vi "Point Shoot Example - MultipleSpectro.vi"(8 "Error in (no error)":errorcluster, 9 "Y":dbl, 10 "X":dbl, 11 "Method":enum16{"init", "run", "end"}(ring)) -> (0 "Error out":errorcluster)   [LabVIEW 2016]
doc: "Example of a measurement VI to be used in the \"Point & Shoot\" tool in Follow Me mode as external VI.\n\nThis example performs multiple bias spectroscopy measurements after each movement.\n\n- Nanonis Programming Interface -"
uses:
  Nanonis Prog Interface.lvlib
panel:
  in  "# Spectro. per point":i32=4
  # "Example of a measurement VI to be used in the \"Point & Shoot\" section of Follow Me mode as external VI.\n\nThis example performs multiple spectroscopy measurement after the movement in the Follow Me mode when Point & Shoot is enabled.\n\nTo use it, set up the bias spectroscopy module to record the desired channels and set all other spectroscopy parameters. Then, set up the experiments on Point & Shoot section to use this VI as \"external VI\".\n \n\"Point & Shoot\" will first (before starting the measurements) call the external VI with the \"init\" method, passing X and Y coordinates of the point.\nThen, for the measurements, the external VI will be called with the \"run\" method.\nAfter the last measurement, the external VI will be called with the \"end\" method."
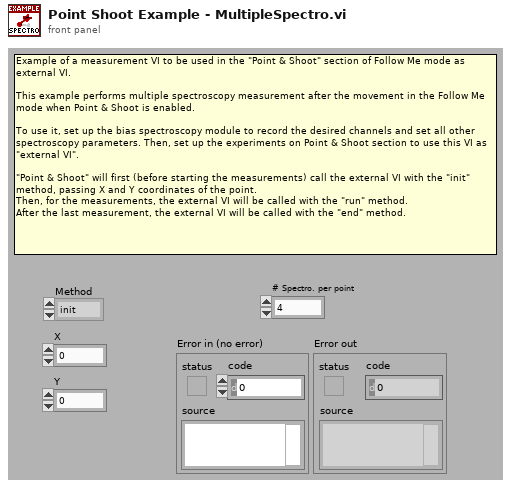
[diagram p1: front panel]
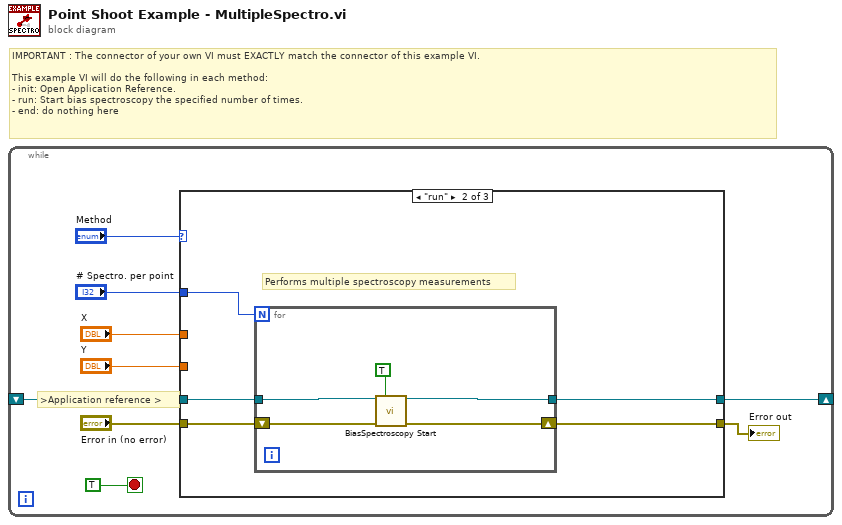
[diagram p0: block diagram]
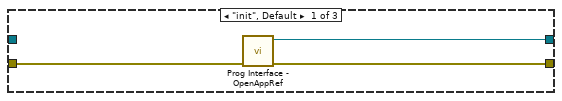
[diagram p2: hidden frame]
diagram:
  # "IMPORTANT : The connector of your own VI must EXACTLY match the connector of this example VI.\n\nThis example VI will do the following in each method:\n- init: Open Application Reference.\n- run: Start bias spectroscopy the specified number of times.\n- end: do nothing here"
  n1 = while {
    shift-right: [w2] -> _
    shift-left: _ -> [w1]
    stop <- TRUE stop-if-true
    # ">Application reference >"
    n2 = case shown="\"run\"" "Method" {
      tunnel: "Error in (no error)" -> [w12 w16 w24]
      tunnel: [w11 w17 w24] -> w6
      tunnel: "X" -> [_ _ _]
      tunnel: "Y" -> [_ _ _]
      tunnel: "# Spectro. per point" -> [_ w15 _]
      tunnel: [w10 w13 w23] -> w2
      tunnel: w1 -> [_ w14 w23]
      frame "init", Default {
        n3 = call <userlib>:"Prog Interface - OpenAppRef.vi"("Error in (no error)"=w12) -> ("Error out"=w11:errorcluster, "Application reference"=w10:refnum<vi>)  [unwired: 5 in]
      }
      frame "run" {
        # "Performs multiple spectroscopy measurements"
        n4 = for {
          N: w15 -> [_]
          shift-right: [w22] -> w17
          shift-left: w16 -> [w21]
          tunnel: w14 -> [w20]
          tunnel: [w19] -> w13
          n5 = call <userlib>:"BiasSpectroscopy Start.vi"("Application ref in"=w20, "Get data (F)"=TRUE ("Get Data (F)"), "Error in (no error)"=w21) -> ("Application ref out"=w19:refnum<vi>, "Error out"=w22:errorcluster)  [unwired: 8 in, 3 out]
        }
      }
      frame "end" {
      }
    }
    "Error out" <- w6
  }
